vi "FlatToRichni_measurementlink_discovery_v1_ResolveServiceWithInformationRequest.vi"(5 "OutputClusterType":T1, 11 "InputCluster":T2) -> (3 "OutputCluster":T1)   [LabVIEW 2024, in "ni.measurementlink.discovery.v1.api.lvlib"]
uses:
  ni.measurementlink.discovery.v1.api.lvlib
  ni_measurementlink_discovery_v1_ResolveServiceWithInformationRequest_Flat.ctl
  ni_measurementlink_discovery_v1_ResolveServiceWithInformationRequest.ctl
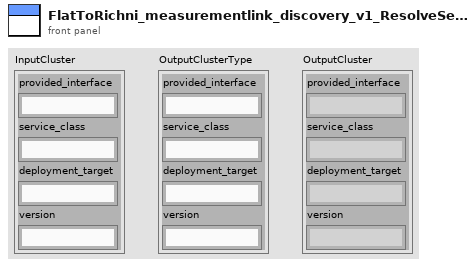
[diagram p1: front panel]
types:
  T1 = typedef "ni.measurementlink.discovery.v1.api.lvlib/ni_measurementlink_discovery_v1_ResolveServiceWithInformationRequest.ctl" = cluster{"provided_interface":string, "service_class":string, "deployment_target":string, "version":string}
  T2 = typedef "ni.measurementlink.discovery.v1.api.lvlib/ni_measurementlink_discovery_v1_ResolveServiceWithInformationRequest_Flat.ctl" = cluster{"provided_interface":string, "service_class":string, "deployment_target":string, "version":string}
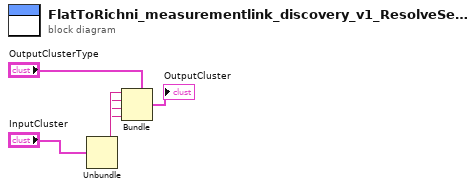
[diagram p0: block diagram]
diagram:
  n1 = Unbundle "Unbundle"("InputCluster") -> ("provided_interface"=w4:string, "service_class"=w3:string, "deployment_target"=w2:string, "version"=w1:string)
  n2 = Bundle "Bundle"(cluster="OutputClusterType", "provided_interface"=w4, "service_class"=w3, "deployment_target"=w2, "version"=w1) -> (→"OutputCluster":T1)
